vi "StateObserver.vi"(4 "L":dbl[](array[numeric])=[2.925, 0.279], 5 "Pb":dbl[](array[numeric])=[0.1281, 0.0001], 6 "Pc":T1=[[0.0, 2.15]], 7 "Pa":T1=[[1.0012, 0.0117], [0.016, 1.0001]], 9 "y[k]":dbl, 10 "u[k]":dbl, 11 "x[k]":dbl[](array[numeric])) -> (1 "y~[k]":dbl, 2 "y^[k]":dbl, 3 "x[k+1]":dbl[](array[numeric]))   [LabVIEW 2016]
uses:
  <vilib>/Analysis/Matrix/Datatypes/RealMatrix.ctl
  <vilib>/Analysis/baseanly.llb/A x Vector.vi
  <vilib>/Analysis/NI_AALBase.lvlib
  <vilib>/Analysis/Matrix/NI_Matrix.lvlib
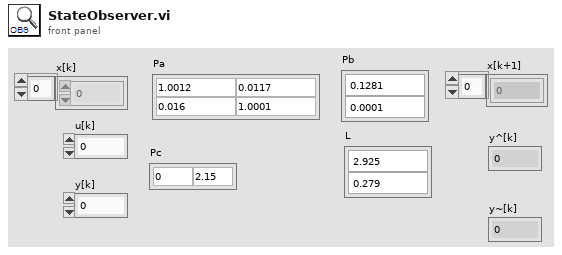
[diagram p1: front panel]
types:
  T1 = typedef "NI_Matrix.lvlib/RealMatrix.ctl" = dbl[][]
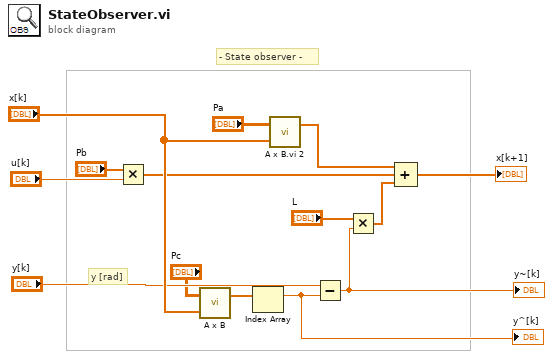
[diagram p0: block diagram]
diagram:
  # "- State observer -"
  # "y [rad]"
  n1 = Multiply ("Multiply 8")(x="Pb", y="u[k]") -> (x*y=w7:dbl[])
  n2 = call-poly <vilib>:"A x B.vi"("Vector"="x[k]", "A"="Pc") -> ("A x Vector"=w2:dbl[])  [unwired: 1 out]
  n3 = Index Array(array=w2) -> (element=w1:dbl)  [unwired: 1 in]
  "y^[k]" <- w1
  n4 = call-poly "A x B.vi 2"("Vector"="x[k]", "A"="Pa") -> ("A x Vector"=w5:dbl[])  [unwired: 1 out]
  n5 = Subtract ("Subtract 2")(x="y[k]", y=w1) -> (x-y=w10:dbl)
  "y~[k]" <- w10
  n6 = Multiply ("Multiply.vi")(x="L", y=w10) -> (x*y=w9:dbl[])
  n7 = Compound Arithmetic op=ADD(w5, w7, w9) -> (→"x[k+1]":dbl[])
